vi "Filter_Evaluator.vi"(7 "Headers and Types":string[][](array[string])=[["Packet Number", "Timestamp", "Source", "Destination", "Protocol", "Length", "Data", "Hex_Data"], ["NUM", "STR", "STR", "STR", "STR", "NUM", "STR", "HEX"]], 8 "Error":errorcluster, 9 "Comparators":T1(array[cluster]), 10 "Boolean Connectors":string[](array[string])=["AND", "OR"], 11 "Prefiltered Data":string[][](array[string])=array1500x8[12000 elements]) -> (0 "Error Out":errorcluster, 2 "Filtered Array":string[][](array[string]), 3 "Prefiltered Data":string[][](array[string]))   [LabVIEW 2025, in "Table_Filtering.lvlib"]
uses:
  Table_Filtering.lvlib
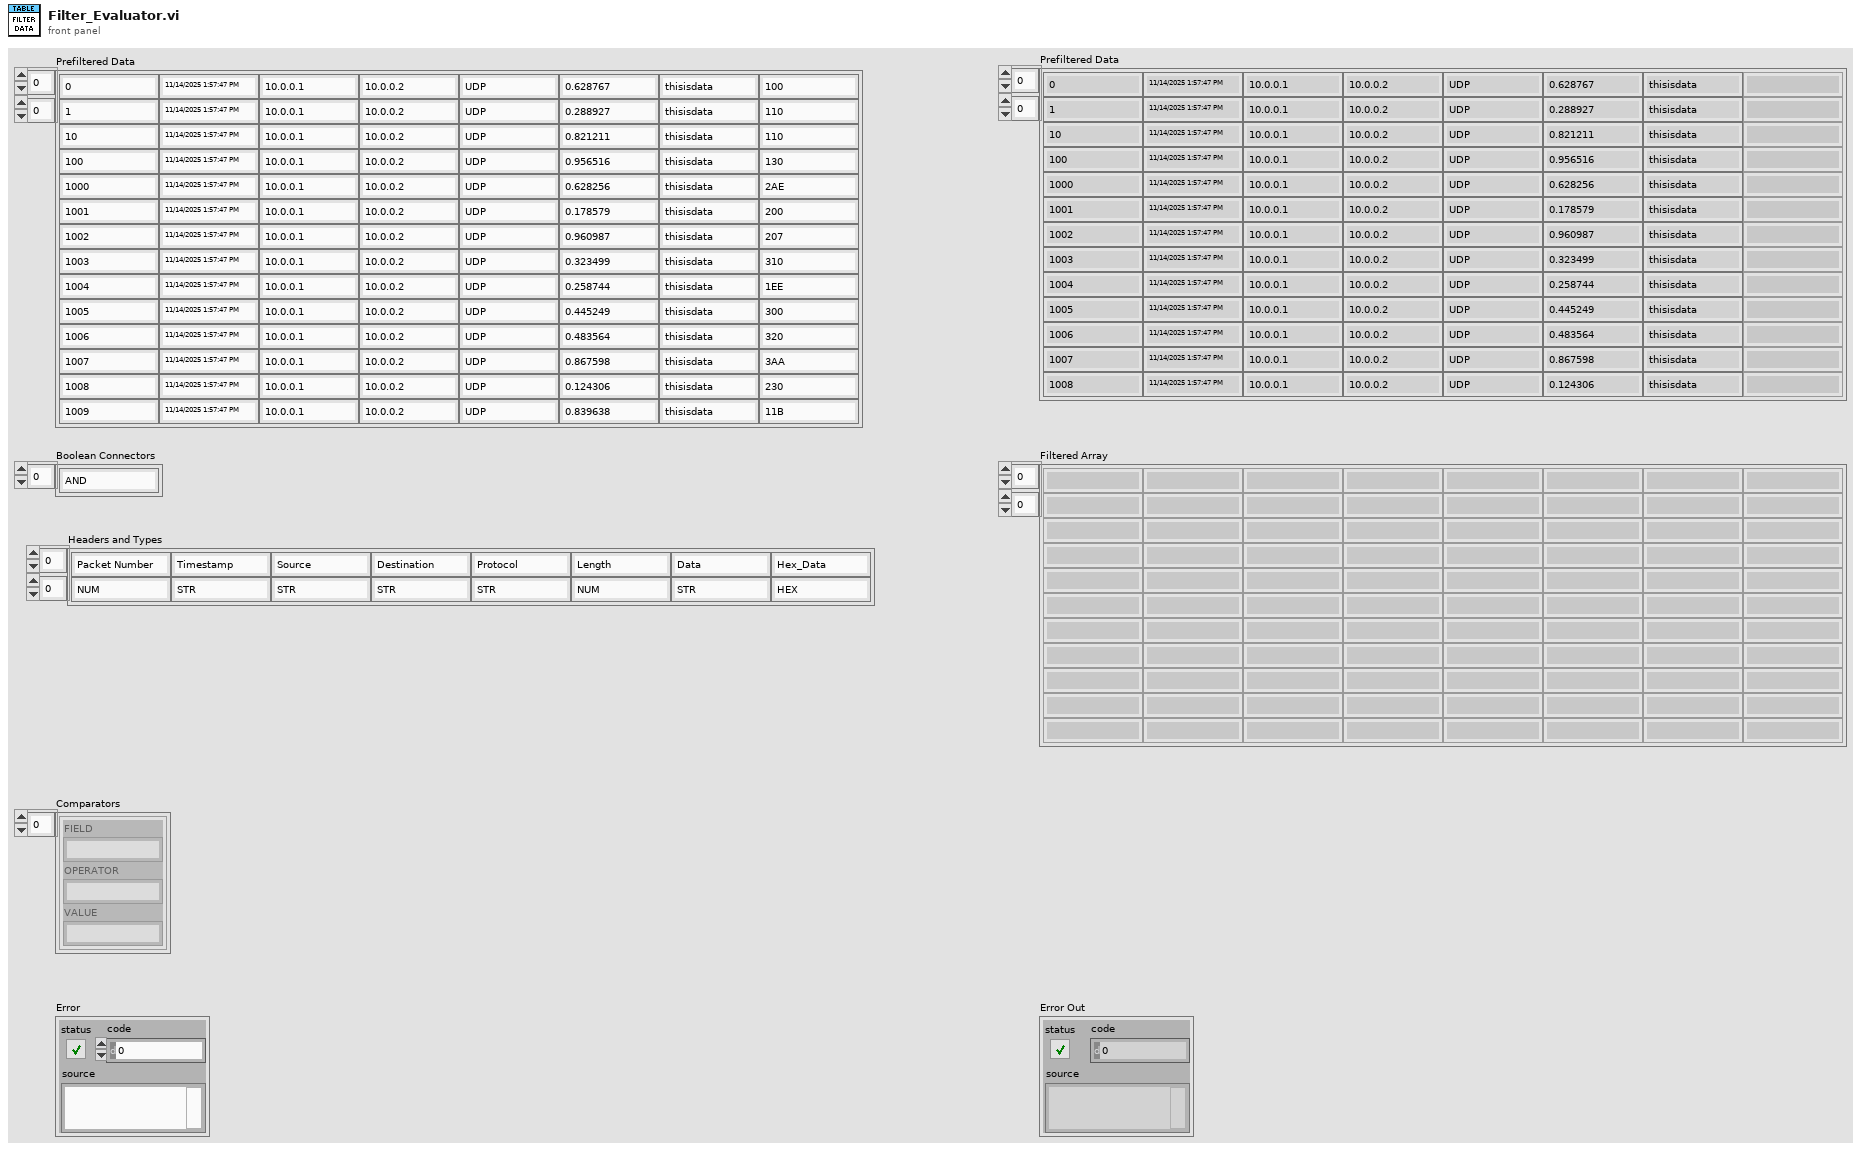
[diagram p1: front panel]
types:
  T1 = cluster{"FIELD":string, "OPERATOR":string, "VALUE":string}[]
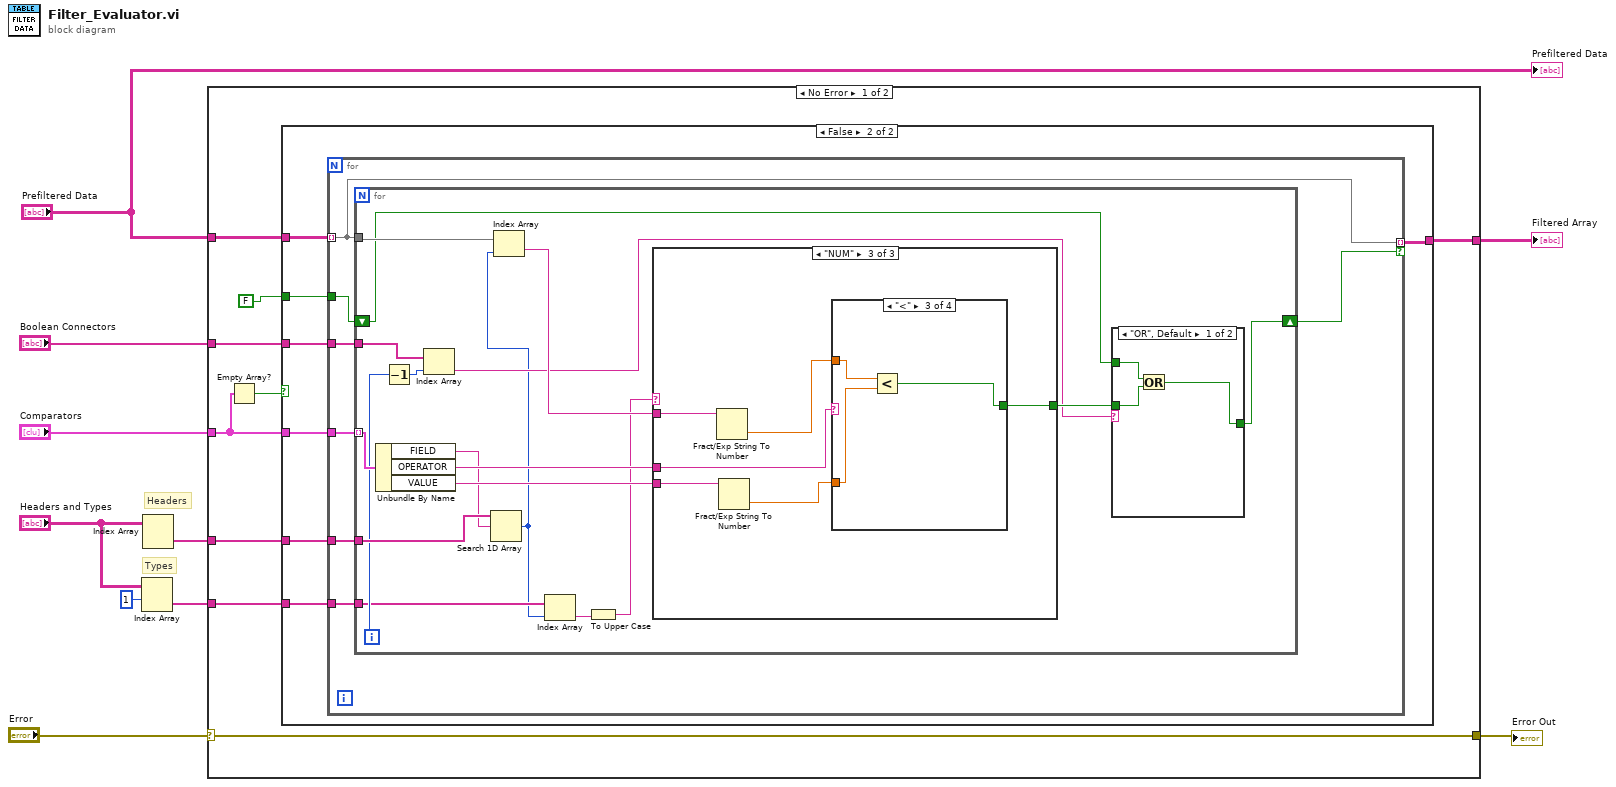
[diagram p0: block diagram]
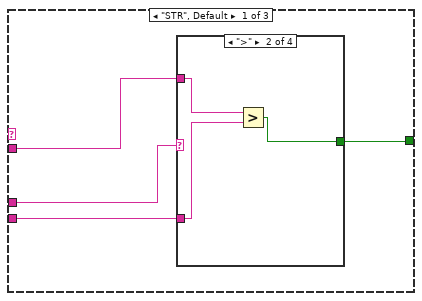
[diagram p3: hidden frame]
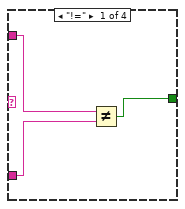
[diagram p4: hidden frame]
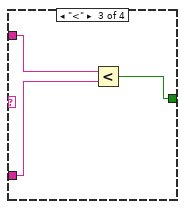
[diagram p5: hidden frame]
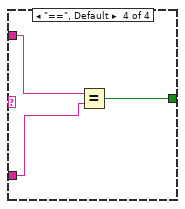
[diagram p6: hidden frame]
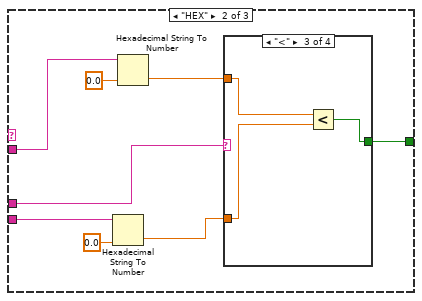
[diagram p7: hidden frame]
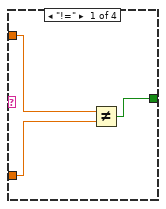
[diagram p8: hidden frame]
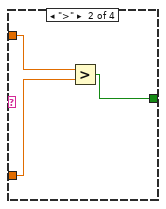
[diagram p9: hidden frame]
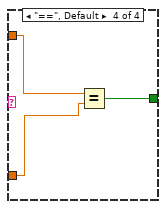
[diagram p10: hidden frame]
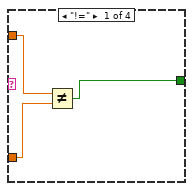
[diagram p11: hidden frame]
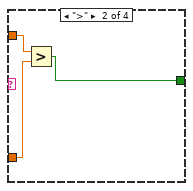
[diagram p12: hidden frame]
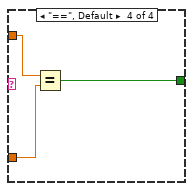
[diagram p13: hidden frame]
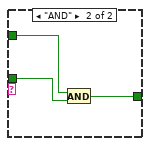
[diagram p14: hidden frame]
diagram:
  # "Types"
  # "Headers"
  n1 = Index Array(array="Headers and Types", index (row)=1) -> (element=w2:string[])  [unwired: 1 in]
  n2 = Index Array(array="Headers and Types") -> (element=w5:string[])  [unwired: 2 in]
  n3 = case shown="No Error" "Error" {
    selector: "Error" -> [w15 w113]
    tunnel: w5 -> [w19 _]
    tunnel: "Boolean Connectors" -> [w18 _]
    tunnel: "Comparators" -> [w12 _]
    tunnel: "Prefiltered Data" -> [w17 _]
    tunnel: [w16 _] -> w10
    tunnel: [w15 w113] -> w7
    tunnel: w2 -> [w11 _]
    frame No Error {
      n4 = Empty Array?(array=w12) -> (empty?=w13:bool)
      n5 = case shown="False" w13 {
        tunnel: w19 -> [_ w27]
        tunnel: FALSE -> [_ w26]
        tunnel: w18 -> [_ w25]
        tunnel: w12 -> [_ w24]
        tunnel: w17 -> [w20 w23]
        tunnel: [w20 w22] -> w16
        tunnel: w11 -> [_ w21]
        frame True {
        }
        frame False {
          n6 = for {
            tunnel: w27 -> [w34]
            tunnel: w24 -> [w33]
            tunnel: w23 -> [w29] mode=indexing
            tunnel: w26 -> [w32]
            tunnel: w25 -> [w31]
            tunnel: [w29] -> w22 mode=indexing if=w30
            tunnel: w21 -> [w28]
            n7 = for {
              tunnel: w34 -> [w50]
              tunnel: w33 -> [w52] mode=indexing
              tunnel: w29 -> [w51]
              shift-right: [w45] -> w30
              shift-left: w32 -> [w46]
              tunnel: w31 -> [w49]
              tunnel: w28 -> [w38]
              i -> [w47]
              n8 = Unbundle By Name(w52) -> ("FIELD"=w39:string, "OPERATOR"=w42:string, "VALUE"=w43:string)
              n9 = Decrement(x=w47) -> (x-1=w48:i32)
              n10 = Index Array(array=w49, index=w48) -> (element=w40:string)
              n11 = Search 1D Array(1D array=w50, element=w39) -> (index of element=w37:i32)  [unwired: 1 in]
              n12 = Index Array(array=w51, index=w37) -> (element=w44:string)
              n13 = Index Array(array=w38, index=w37) -> (element=w36:string)
              n14 = To Upper Case(1:w36) -> (0:w35:string)
              n15 = case shown="\"NUM\"" w35 {
                tunnel: w44 -> [w56 w76 w94]
                tunnel: w43 -> [w53 w72 w90]
                tunnel: w42 -> [w55 w74 w93]
                tunnel: [w54 w73 w92] -> w41
                frame "STR", Default {
                  n16 = case shown="\">\"" w55 {
                    tunnel: w56 -> [w58 w62 w65 w66]
                    tunnel: w53 -> [w57 w61 w64 w68]
                    tunnel: [w59 w60 w63 w67] -> w54
                    frame "!=" {
                      n17 = Not Equal?(x=w58, y=w57) -> (x != y?=w59:bool)
                    }
                    frame ">" {
                      n18 = Greater?(x=w62, y=w61) -> (0:w60:bool)
                    }
                    frame "<" {
                      n19 = Less?(x=w65, y=w64) -> (x < y?=w63:bool)
                    }
                    frame "==", Default {
                      n20 = Equal?(x=w66, y=w68) -> (x = y?=w67:bool)
                    }
                  }
                }
                frame "HEX" {
                  n21 = Hexadecimal String To Number(string=w72, default (0uL)=0.0) -> (number=w69:dbl)  [unwired: 1 in, 1 out]
                  n22 = Hexadecimal String To Number(string=w76, default (0uL)=0.0) -> (number=w75:dbl)  [unwired: 1 in, 1 out]
                  n23 = case shown="\"<\"" w74 {
                    tunnel: w75 -> [w78 w82 w85 w86]
                    tunnel: w69 -> [w77 w81 w84 w88]
                    tunnel: [w79 w80 w83 w87] -> w73
                    frame "!=" {
                      n24 = Not Equal?(x=w78, y=w77) -> (x != y?=w79:bool)
                    }
                    frame ">" {
                      n25 = Greater?(x=w82, y=w81) -> (0:w80:bool)
                    }
                    frame "<" {
                      n26 = Less?(x=w85, y=w84) -> (x < y?=w83:bool)
                    }
                    frame "==", Default {
                      n27 = Equal?(x=w86, y=w88) -> (x = y?=w87:bool)
                    }
                  }
                }
                frame "NUM" {
                  n28 = Fract/Exp String To Number(string=w94) -> (number=w91:dbl)  [unwired: 3 in, 1 out]
                  n29 = Fract/Exp String To Number(string=w90) -> (number=w89:dbl)  [unwired: 3 in, 1 out]
                  n30 = case shown="\"<\"" w93 {
                    tunnel: w89 -> [w96 w100 w103 w106]
                    tunnel: [w97 w99 w102 w105] -> w92
                    tunnel: w91 -> [w95 w98 w101 w104]
                    frame "!=" {
                      n31 = Not Equal?(x=w95, y=w96) -> (x != y?=w97:bool)
                    }
                    frame ">" {
                      n32 = Greater?(x=w98, y=w100) -> (0:w99:bool)
                    }
                    frame "<" {
                      n33 = Less?(x=w101, y=w103) -> (x < y?=w102:bool)
                    }
                    frame "==", Default {
                      n34 = Equal?(x=w104, y=w106) -> (x = y?=w105:bool)
                    }
                  }
                }
              }
              n35 = case shown="\"OR\", Default" w40 {
                tunnel: w46 -> [w108 w112]
                tunnel: [w109 w111] -> w45
                tunnel: w41 -> [w107 w110]
                frame "OR", Default {
                  n36 = Or(x=w108, y=w107) -> (x .or. y?=w109:bool)
                }
                frame "AND" {
                  n37 = And(x=w112, y=w110) -> (x .and. y?=w111:bool)
                }
              }
            }
          }
        }
      }
    }
    frame Error {
    }
  }
  "Filtered Array" <- w10
  "Error Out" <- w7
  "Prefiltered Data" <- "Prefiltered Data"
